vi "Simulated-PowerModule_GetAttributes.vi"(0 "reference in":refnum<class "Simulated-PowerModule.lvclass">, 5 "OnlyGetDvrReference(False)":bool, 11 "Error In":errorcluster) -> (4 "reference out":refnum<class "Simulated-PowerModule.lvclass">, 6 "Data":T1={"JSON Config Path"=path "", "Configuration"={"IP Address"=""}, "connected"=FALSE, "reserved"=FALSE, "energized"=FALSE, "output enabled"=FALSE, "Mode"=193, "Range"={"Current Max (A)"=0.0, "Current Min (A)"=0.0, "Voltage Max (V)"=0.0, "Voltage Min (V)"=0.0}, "Slew Rates"={"Current Decrease (A/sec)"=0.0, "Current Increase (A/sec)"=0.0, "Voltage Decrease (V/sec)"=0.0, "Voltage Increase (V/sec)"=0.0, "Resistance Decrease (Ohm/sec)"=0.0, "Resistance Increase (Ohm/sec)"=0.0}, "Setpoints"={"voltage"=0.0, "current"=0.0, "resistance"=0.0}, "Measurements"={"voltage"=0.0, "current"=0.0, "resistance"=0.0}, "Limits"={"Current Max (A)"=0.0, "Current Min (A)"=0.0, "Voltage Max (V)"=0.0, "Voltage Min (V)"=0.0, "Power Max (W)"=0.0, "Power Min (W)"=0.0}, "active faults"=[], "fault"=FALSE, "profile"=[], "step dt"=0} {"Mode" items=["CONSTANT VOLTAGE (V+R)"=1, "CONSTANT CURRENT (I)"=2]}, 10 "DataRef":refnum<data-value>, 15 "Error Out":errorcluster)   [LabVIEW 2023, in "Simulated-PowerModule.lvlib" / "Simulated-PowerModule.lvclass"]
uses:
  Simulated-PowerModule.lvclass
  protected/ObjectAttributes.ctl
  Configuration.ctl
  Mode.ctl
  builds/PowerModuleInterface/PowerModuleInterface.lvlibp/Classes/PowerModule_interface/Range.ctl
  builds/PowerModuleInterface/PowerModuleInterface.lvlibp/Classes/PowerModule_interface/Slew Rates.ctl
  builds/PowerModuleInterface/PowerModuleInterface.lvlibp/Classes/PowerModule_interface/Limits.ctl
  Simulated-PowerModule.lvclass/Simulated-PowerModule.ctl
  builds/PowerModuleInterface/PowerModuleInterface.lvlibp/Classes/PowerModule_interface/PowerModuleInterface.lvclass
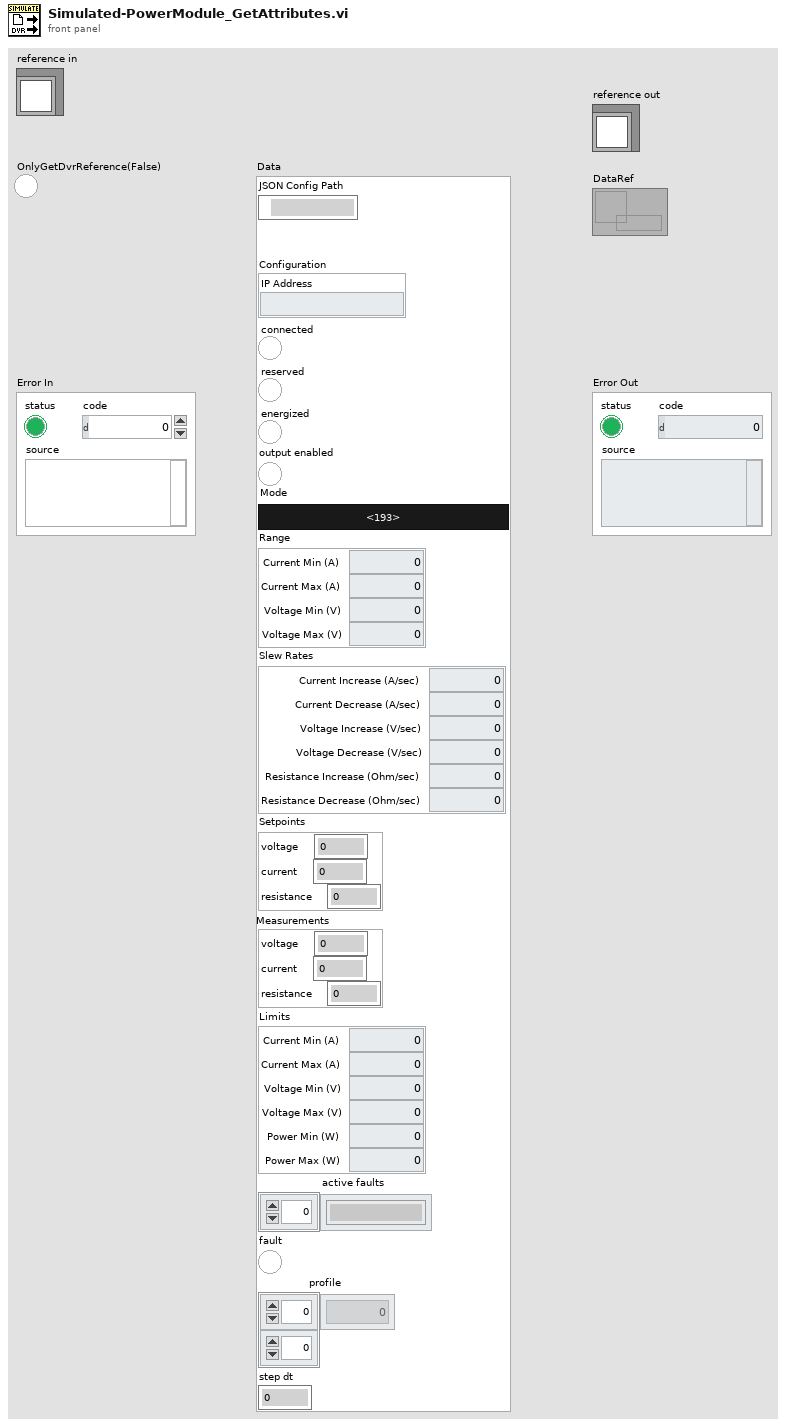
[diagram p1: front panel]
types:
  T1 = typedef "Simulated-PowerModule.lvlib/Simulated-PowerModule.lvclass/ObjectAttributes.ctl" = cluster{"JSON Config Path":path, "Configuration":T2, "connected":bool, "reserved":bool, "energized":bool, "output enabled":bool, "Mode":T3, "Range":T4, "Slew Rates":T5, "Setpoints":cluster{"voltage":dbl, "current":dbl, "resistance":dbl}, "Measurements":cluster{"voltage":dbl, "current":dbl, "resistance":dbl}, "Limits":T6, "active faults":string[], "fault":bool, "profile":dbl[][], "step dt":i64}
  T2 = typedef "Simulated-PowerModule.lvlib/Simulated-PowerModule.lvclass/Configuration.ctl" = cluster{"IP Address":string}
  T3 = typedef "Simulated-PowerModule.lvlib/Simulated-PowerModule.lvclass/Mode.ctl" = u16
  T4 = typedef "PowerModuleInterface.lvlibp/PowerModuleInterface.lvclass/Range.ctl" = cluster{"Current Max (A)":dbl, "Current Min (A)":dbl, "Voltage Max (V)":dbl, "Voltage Min (V)":dbl}
  T5 = typedef "PowerModuleInterface.lvlibp/PowerModuleInterface.lvclass/Slew Rates.ctl" = cluster{"Current Decrease (A/sec)":dbl, "Current Increase (A/sec)":dbl, "Voltage Decrease (V/sec)":dbl, "Voltage Increase (V/sec)":dbl, "Resistance Decrease (Ohm/sec)":dbl, "Resistance Increase (Ohm/sec)":dbl}
  T6 = typedef "PowerModuleInterface.lvlibp/PowerModuleInterface.lvclass/Limits.ctl" = cluster{"Current Max (A)":dbl, "Current Min (A)":dbl, "Voltage Max (V)":dbl, "Voltage Min (V)":dbl, "Power Max (W)":dbl, "Power Min (W)":dbl}
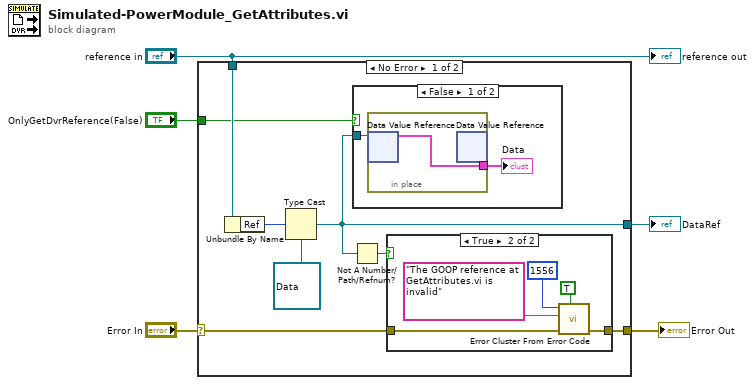
[diagram p0: block diagram]
diagram:
  n1 = case shown="No Error" "Error In" {
    selector: "Error In" -> [w7 w23]
    tunnel: "reference in" -> [w13 _]
    tunnel: [w12 _] -> w4
    tunnel: "OnlyGetDvrReference(False)" -> [w11 _]
    tunnel: [w6 w23] -> w1
    frame No Error {
      n2 = Unbundle By Name(w13) -> ("Ref"=w10:u32)
      n3 = Type Cast(type=refnum<data-value> refnum, x=w10) -> (*(type *) &x=w12:refnum<data-value>)
      n4 = Not A Number/Path/Refnum?(number/path/refnum=w12) -> (NaN/Path/Refnum?=w9:bool)
      n5 = case shown="False" w11 {
        tunnel: w12 -> [w21 _]
        frame False {
          n6 = in-place {
            in-place-border: [w22] -> w20
            n7 = in-place-dvr #1(w21) -> (w22:T1)  [unwired: 1 out]
            n8 = in-place-dvr #1() -> ()  [unwired: 1 in, 2 out]
          }
          "Data" <- w20
        }
        frame True {
        }
      }
      n9 = case shown="True" w9 {
        tunnel: w7 -> [w14 w17]
        tunnel: [w14 w16] -> w6
        frame False {
        }
        frame True {
          n10 = call <vilib>:"Error Cluster From Error Code.vi"("show call chain? (False)"=TRUE, "error in (no error)"=w17, "error message (\"\")"="The GOOP reference at GetAttributes.vi is invalid" ("source"), "error code (0)"=1556 ("code")) -> ("error out"=w16:errorcluster)  [unwired: 5 in]
        }
      }
    }
    frame Error {
    }
  }
  "DataRef" <- w4
  "Error Out" <- w1
  "reference out" <- "reference in"
